vi "fgv_DSP_config.vi"(7 "cmd":T2, 8 "error in (no error)":errorcluster, 10 "DSP Config LV IN":T1={"Port"="TCPIP0::192.168.0.14::HISLIP0::INSTR", "OVP Level"=0.0, "OCP Level"=0.0, "Current"=0.0, "Voltage"=0.0} {"OCP Level" format="%#_13g"; "OVP Level" format="%#_13g"}, 11 "DSP Config HV IN":T1={"Port"="TCPIP0::192.168.0.14::HISLIP0::INSTR", "OVP Level"=0.0, "OCP Level"=0.0, "Current"=0.0, "Voltage"=0.0} {"OCP Level" format="%#_13g"; "OVP Level" format="%#_13g"}) -> (0 "error out":errorcluster, 2 "DSP Config LV OUT":T1={"Port"="TCPIP0::192.168.0.14::HISLIP0::INSTR", "OVP Level"=0.0, "OCP Level"=0.0, "Current"=0.0, "Voltage"=0.0} {"OCP Level" format="%#_13g"; "OVP Level" format="%#_13g"}, 3 "DSP Config HV OUT":T1={"Port"="TCPIP0::192.168.0.14::HISLIP0::INSTR", "OVP Level"=0.0, "OCP Level"=0.0, "Current"=0.0, "Voltage"=0.0} {"OCP Level" format="%#_13g"; "OVP Level" format="%#_13g"})   [LabVIEW 2019]
uses:
  _ctrl/rw.ctl
  _ctrl/DSP_config.ctl
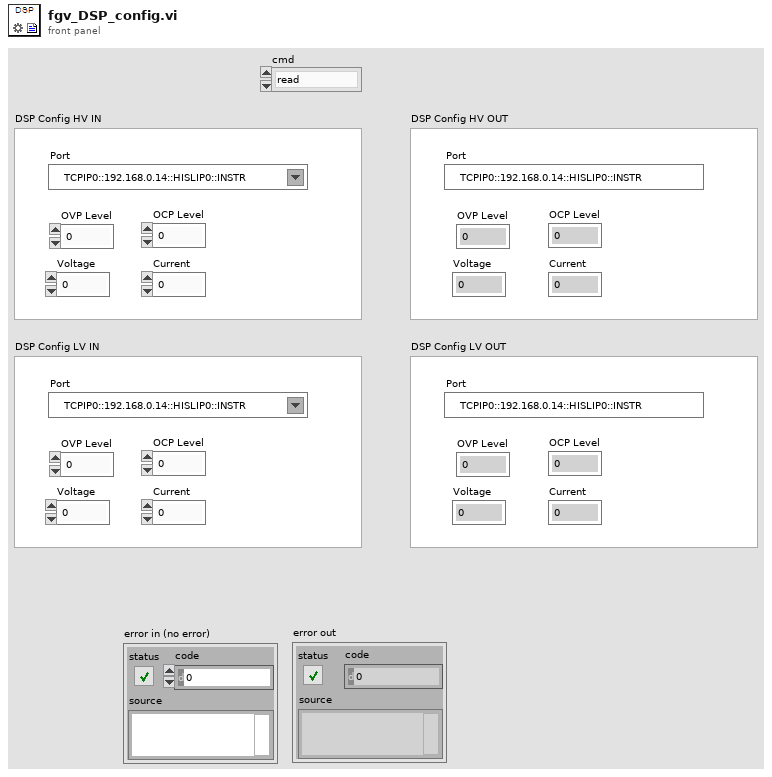
[diagram p1: front panel]
types:
  T1 = typedef "DSP_config.ctl" = cluster{"Port":refnum<visa-resource-name>, "OVP Level":dbl, "OCP Level":dbl, "Current":dbl, "Voltage":dbl}
  T2 = typedef "rw.ctl" = enum16{"read", "write"}
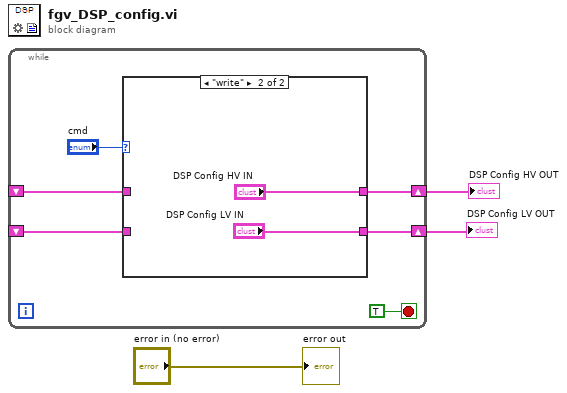
[diagram p0: block diagram]
diagram:
  n1 = while {
    shift-right: [w7] -> w3
    shift-left: _ -> [w6]
    shift-right: [w5] -> w1
    shift-left: _ -> [w4]
    stop <- TRUE stop-if-true
    n2 = case shown="\"write\"" "cmd" {
      tunnel: [w11 "DSP Config HV IN"] -> w7
      tunnel: w6 -> [w11 _]
      tunnel: [w10 "DSP Config LV IN"] -> w5
      tunnel: w4 -> [w10 _]
      frame "read", Default {
      }
      frame "write" {
      }
    }
  }
  "DSP Config HV OUT" <- w3
  "DSP Config LV OUT" <- w1
  "error out" <- "error in (no error)"
